vi "rename channel test.vi"() -> ()   [LabVIEW 2013, in "UI reference module tests.lvlib"]
uses:
  UI reference module tests.lvlib
  <vilib>/NI/Tag Bus/tag/tag descriptor.lvclass
  module/configuration/UI Reference configuration.lvclass
  <vilib>/NI/Configuration Framework/serializable configuration/NISE_CEF_serializable configuration.lvclass
panel:
  out "rename success":bool
  out "no err":errorcluster
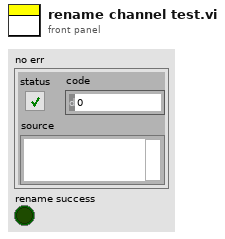
[diagram p1: front panel]
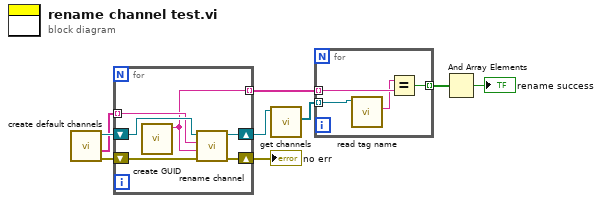
[diagram p0: block diagram]
diagram:
  n1 = call "create default channels.vi"() -> ("error out"=w1:errorcluster, "names"=w2:string[], "module"=w3:refnum<class "UI Reference configuration.lvclass">)  [unwired: 7 in, 2 out]
  n2 = for {
    tunnel: w2 -> [w11] mode=indexing
    shift-right: [w12] -> w9
    shift-left: w3 -> [w15]
    shift-right: [w13] -> w7
    shift-left: w1 -> [w14]
    tunnel: [w10] -> w8 mode=indexing
    n3 = call <vilib>:"create GUID.vi"() -> ("uuid"=w10:string)  [unwired: 11 in]
    n4 = call "rename channel.vi"("error in"=w14, "new name"=w10, "old name"=w11, "UI Reference configuration in"=w15) -> ("error out"=w13:errorcluster, "UI Reference configuration out"=w12:refnum<class "UI Reference configuration.lvclass">)  [unwired: 6 in]
  }
  "no err" <- w7
  n5 = call-dynamic "get channels.vi"("UI Reference configuration in"=w9) -> ("channels"=w6:refnum<class "TBM channel.lvclass">[])  [unwired: 9 in, 1 out]
  n6 = for {
    tunnel: w8 -> [w18] mode=indexing
    tunnel: w6 -> [w19] mode=indexing
    tunnel: [w16] -> w5 mode=indexing
    n7 = call <vilib>:"read tag name.vi"("system tag in"=w19) -> ("name"=w17:string)  [unwired: 8 in, 2 out]
    n8 = Equal?(x=w17, y=w18) -> (x = y?=w16:bool)
  }
  n9 = And Array Elements(Boolean array=w5) -> (logical AND=→"rename success":bool)
